vi "niDTS DUT to BT DUT.vi"(9 "error in":errorcluster, 10 "Dut Handle":T2) -> (1 "error out":errorcluster, 2 "BT Dut Handle":T1)   [LabVIEW 2015, in "niDTS BT.lvlib" / "niDTS BT Dut.lvclass"]
uses:
  niDTS BT Dut.lvclass
  Framework/Dut/Includes/niDTS Dut INC Handle.ctl
  Framework/Dut/Objects/BASE_class/niDTS Dut.lvclass
  Includes/niDTS BT Dut INC Handle.ctl
  niDTS BT.lvlib
  Framework/niDTS Framework.lvlib
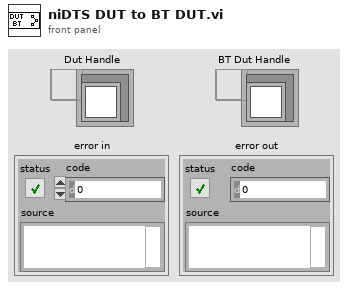
[diagram p1: front panel]
types:
  T1 = typedef "niDTS BT.lvlib/niDTS BT Dut INC Handle.ctl" = refnum<data-value>
  T2 = typedef "niDTS Framework.lvlib/niDTS Dut INC Handle.ctl" = refnum<data-value>
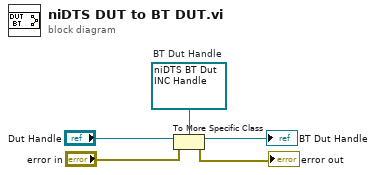
[diagram p0: block diagram]
diagram:
  w1 = T1 refnum  # BT Dut Handle
  n1 = To More Specific Class(target class=w1, reference="Dut Handle", error in="error in") -> (specific class reference=→"BT Dut Handle":T1, error out=→"error out":errorcluster)
